vi "WORD_To_Float.vi"(10 "second_Word":u16, 11 "first_Word":u16) -> (3 "output_Float":sgl)   [LabVIEW 2023, in "Drive.lvlib"]
uses:
  Drive.lvlib
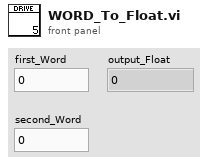
[diagram p1: front panel]
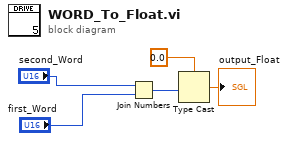
[diagram p0: block diagram]
diagram:
  n1 = Join Numbers(hi="second_Word", lo="first_Word") -> ((hi.lo)=w2:u32)
  n2 = Type Cast(type=sgl 0.0, x=w2) -> (*(type *) &x=→"output_Float":sgl)
